vi "ConfigDevice.vi"(8 "error in (no error)":errorcluster, 11 "NHRDCModel in":refnum<class "NHRDCPowerModel.lvclass">) -> (0 "error out":errorcluster, 3 "NHRDCModel out":refnum<class "NHRDCPowerModel.lvclass">)   [LabVIEW 2018, in "AcPwrPlugins.lvlib" / "NHRDCPowerModel.lvclass"]
doc: "This VI configures all the properties set by the user through the INI file or the Properties Dialog box."
uses:
  NHRDCPowerModel.lvclass
  NHRDCPowerModel.lvclass/NHRDCPowerModel.ctl
  Database/DatabaseBaseClass/DatabaseBaseClass.lvclass
  <vilib>/addons/database/NI_Database_API.lvlib
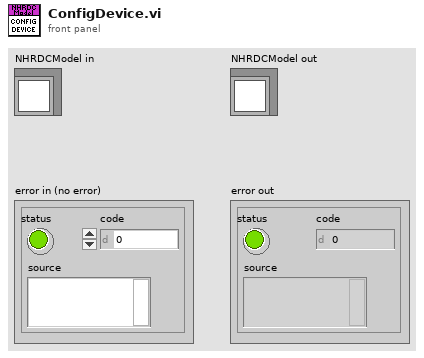
[diagram p1: front panel]
types:
  T1 = typedef "AcPwrPlugins.lvlib/NHRDCPower.lvclass/Device(s)Settings.ctl" = cluster{"MeasName":string, "Modules":T2}
  T2 = typedef "AcPwrPlugins.lvlib/NHRDCPower.lvclass/Modules.ctl" = cluster{"Handle":string, "Name":string, "id query (Yes)":bool, "reset device (Yes)":bool, "Connected":bool, "Initial Battery Detect Voltage (0)":dbl, "SafetySettings":cluster{"SetWatchDog?":bool, "Voltage (V)":dbl, "Current (A)":dbl, "Power (W)":dbl, "Voltage Delay (s)":dbl, "Current Delay (s)":dbl, "Power Delay (s)":dbl}, "Options String":string, "Aperture Time (s)":dbl, "operating state (Off)":i32, "OutputSettings":cluster{"Voltage (V)":dbl, "Current (A)":dbl, "Resistance (Ohms)":dbl, "Power (W)":dbl, "Enable Voltage":bool, "Enable Current":bool, "Enable Resistance":bool, "Enable Power":bool, "Macro After Step Delay  (s)":dbl, "Wait Value (V, A, W)":dbl, "Enable Wait":bool, "Wait on Value":i32}, "SlewRate":cluster{"Set Voltage Rate V/S":dbl, "Set Current Rate A/S":dbl, "Set Resistance Rate R/S":dbl, "Set Power Rate W/S":dbl}, "Macro":cluster{"Save Macro?":bool, "Load Macro From File?":bool, "Run Macro Continuously?":bool, "Use Macros?":bool, "Load Macro File Path":path, "Save Macro File Path":string}, "Regulation Gain (1=100%)":dbl, "UpdatingOntheFly":bool}[]
  T3 = typedef "AcPwrShared.lvlib/Database Settings.ctl" = cluster{"Data Source":string, "ICDAS to Model Table":string, "Model to ICDAS Table":string}
  T4 = typedef "NI_Database_API.lvlib/Conn ObjectReference.ctl" = refnum<k1>
  T5 = cluster{"Handle":string, "Name":string, "id query (Yes)":bool, "reset device (Yes)":bool, "Connected":bool, "Initial Battery Detect Voltage (0)":dbl, "SafetySettings":cluster{"SetWatchDog?":bool, "Voltage (V)":dbl, "Current (A)":dbl, "Power (W)":dbl, "Voltage Delay (s)":dbl, "Current Delay (s)":dbl, "Power Delay (s)":dbl}, "Options String":string, "Aperture Time (s)":dbl, "operating state (Off)":i32, "OutputSettings":cluster{"Voltage (V)":dbl, "Current (A)":dbl, "Resistance (Ohms)":dbl, "Power (W)":dbl, "Enable Voltage":bool, "Enable Current":bool, "Enable Resistance":bool, "Enable Power":bool, "Macro After Step Delay  (s)":dbl, "Wait Value (V, A, W)":dbl, "Enable Wait":bool, "Wait on Value":i32}, "SlewRate":cluster{"Set Voltage Rate V/S":dbl, "Set Current Rate A/S":dbl, "Set Resistance Rate R/S":dbl, "Set Power Rate W/S":dbl}, "Macro":cluster{"Save Macro?":bool, "Load Macro From File?":bool, "Run Macro Continuously?":bool, "Use Macros?":bool, "Load Macro File Path":path, "Save Macro File Path":string}, "Regulation Gain (1=100%)":dbl, "UpdatingOntheFly":bool}
  T6 = cluster{string, "Voltage (V)":dbl, "Current (A)":dbl, "Resistance (Ohms)":dbl, "Power (W)":dbl, "Set Voltage Rate V/S":dbl, "Set Current Rate A/S":dbl, "Set Resistance Rate R/S":dbl, "Set Power Rate W/S":dbl, "Initial Battery Detect Voltage (0)":dbl, "Voltage (V)":dbl, "Voltage Delay (s)":dbl, "Current (A)":dbl, "Current Delay (s)":dbl, "Power (W)":dbl, "Power Delay (s)":dbl, "seconds since 1Jan1904":timestamp, bool, "current time":timestamp, "Measurement Refresh Time (ms)":u32}
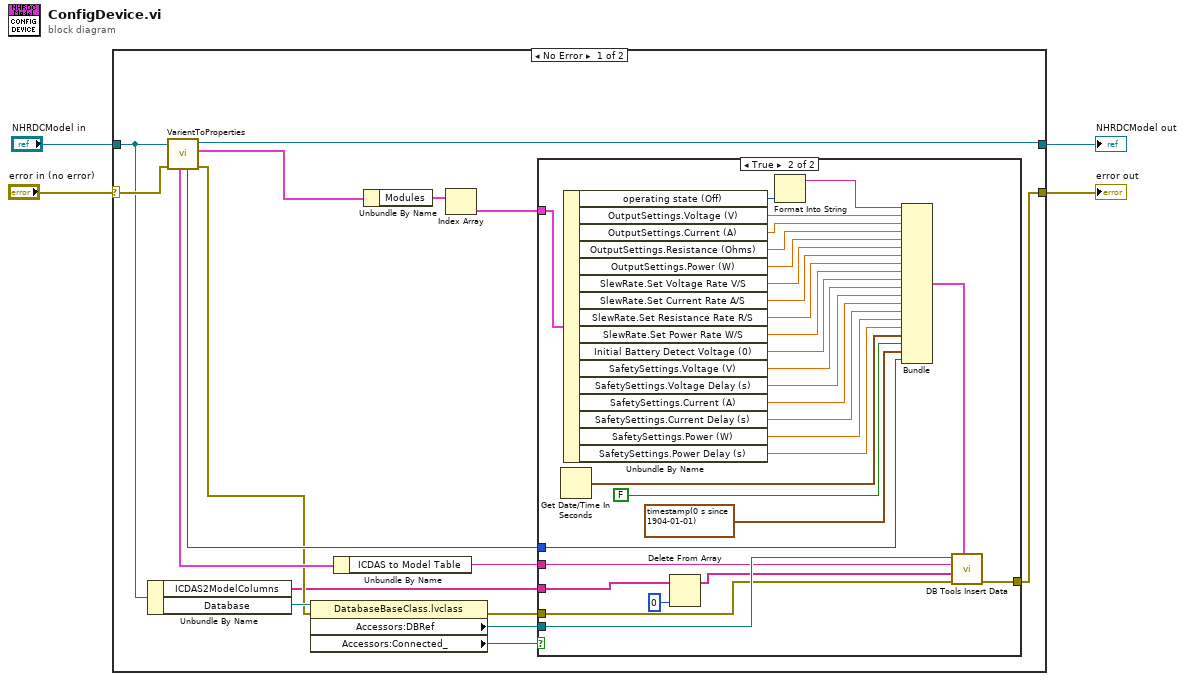
[diagram p0: block diagram]
diagram:
  n1 = case shown="No Error" "error in (no error)" {
    selector: "error in (no error)" -> [w20 w52]
    tunnel: "NHRDCModel in" -> [w19 w53]
    tunnel: [w14 w53] -> w2
    tunnel: [w5 w52] -> w1
    frame No Error {
      n2 = Unbundle By Name(w19) -> ("ICDAS2ModelColumns"=w7:string[], "Database"=w18:refnum<class "DatabaseBaseClass.lvclass">)
      n3 = call "VarientToProperties.vi"("error in (no error)"=w20, "AcPwrPlugins.lvlib:NHRDCModel.lvclass"=w19) -> ("error out"=w9:errorcluster, "Device(s)Settings"=w16:T1, "AcPwrPlugins.lvlib:NHRDCModel.lvclass"=w14:refnum<class "NHRDCPowerModel.lvclass">, "Measurement Refresh Time (ms)"=w10:u32, "Database Settings"=w17:T3)  [unwired: 4 in, 1 out]
      n4 = property class="DatabaseBaseClass.lvclass"(reference=w18, error in=w9) -> (error out=w8:errorcluster, "Accessors:DBRef"=w6:T4, "Accessors:Connected_"=w13:bool)  [unwired: 1 out]
      n5 = Unbundle By Name(w17) -> ("ICDAS to Model Table"=w11:string)
      n6 = Unbundle By Name(w16) -> ("Modules"=w15:T2)
      n7 = Index Array(array=w15) -> (element=w12:T5)  [unwired: 1 in]
      n8 = case shown="True" w13 {
        tunnel: w12 -> [_ w51]
        tunnel: w11 -> [_ w25]
        tunnel: w10 -> [_ w30]
        tunnel: w8 -> [w21 w23]
        tunnel: w7 -> [_ w28]
        tunnel: w6 -> [_ w26]
        tunnel: [w21 w22] -> w5
        frame False {
        }
        frame True {
          n9 = Get Date/Time In Seconds() -> (seconds since 1Jan1904=w33:timestamp)
          n10 = Unbundle By Name(w51) -> ("operating state (Off)"=w50:i32, "OutputSettings.Voltage (V)"=w48:dbl, "OutputSettings.Current (A)"=w47:dbl, "OutputSettings.Resistance (Ohms)"=w46:dbl, "OutputSettings.Power (W)"=w45:dbl, "SlewRate.Set Voltage Rate V/S"=w44:dbl, "SlewRate.Set Current Rate A/S"=w43:dbl, "SlewRate.Set Resistance Rate R/S"=w42:dbl, "SlewRate.Set Power Rate W/S"=w41:dbl, "Initial Battery Detect Voltage (0)"=w40:dbl, "SafetySettings.Voltage (V)"=w39:dbl, "SafetySettings.Voltage Delay (s)"=w38:dbl, "SafetySettings.Current (A)"=w37:dbl, "SafetySettings.Current Delay (s)"=w36:dbl, "SafetySettings.Power (W)"=w35:dbl, "SafetySettings.Power Delay (s)"=w34:dbl)
          n11 = Delete From Array(array=w28, index=0) -> (array with subset deleted=w24:string[])  [unwired: 1 in, 1 out]
          n12 = Format Into String(w50) -> (resulting string=w49:string)  [unwired: 3 in, 1 out]
          n13 = Bundle(w49, "Voltage (V)"=w48, "Current (A)"=w47, "Resistance (Ohms)"=w46, "Power (W)"=w45, "Set Voltage Rate V/S"=w44, "Set Current Rate A/S"=w43, "Set Resistance Rate R/S"=w42, "Set Power Rate W/S"=w41, "Initial Battery Detect Voltage (0)"=w40, "Voltage (V)"=w39, "Voltage Delay (s)"=w38, "Current (A)"=w37, "Current Delay (s)"=w36, "Power (W)"=w35, "Power Delay (s)"=w34, "seconds since 1Jan1904"=w33, FALSE, "current time"=timestamp(0 s since 1904-01-01), "Measurement Refresh Time (ms)"=w30) -> (w29:T6)  [unwired: 1 in]
          n14 = call <vilib>:"DB Tools Insert Data.vi"("data"=w29, "error in (no error)"=w23, "columns"=w24, "table"=w25, "connection reference"=w26) -> ("error out"=w22:errorcluster)  [unwired: 5 in, 1 out]
        }
      }
    }
    frame Error {
    }
  }
  "error out" <- w1
  "NHRDCModel out" <- w2
